vi "PreTell.vi"(8 "TellOriginEnum":T1, 9 "ListenerAlias":string, 10 "Message":refnum<class "Msg.lvclass">, 11 "Actor":refnum<class "Actor.lvclass">) -> (2 "Message":refnum<class "Msg.lvclass">)   [LabVIEW 2020, in "jettl.lvlib"]
uses:
  jettl.lvlib
  Origin.ctl
  Lifecycle.ctl
  Metadata.ctl
  Actor/Actor.lvclass
  Msg/Msg.lvclass
  Metadata/Metadata.lvclass
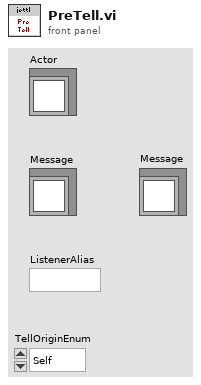
[diagram p1: front panel]
types:
  T1 = typedef "jettl.lvlib/Origin.ctl" = enum16{"Self", "Parent", "Child"}
  T2 = typedef "jettl.lvlib/Metadata.ctl" = cluster{"ListenerAlias":string, "TellerAlias":string, "Lifecycle":T3, "Origin":T1, "AbsoluteTime":timestamp, "RelativeTime":dbl, "Metadata":refnum<class "Metadata.lvclass">}
  T3 = typedef "jettl.lvlib/Lifecycle.ctl" = enum16{"Initializing", "SettingUp", "Starting", "Running", "Stopping", "TearingDown", "Terminated"}
  T4 = typedef "jettl.lvlib/Base.ctl" = cluster{"Lifecycle":T3, "SelfUnified":T5, "ParentUnified":T5, "ChildUnifiedMap":T7}
  T5 = typedef "jettl.lvlib/Unified.ctl" = cluster{"Alias":string, "MsgSet":T6, "Root":bool, "Leaf":bool, "MsgDVREvent":refnum<user-event>, "EventRegRef":refnum<event-registration>, "PreSetupQueue":refnum<queue>, "BeginSetupQueue":refnum<queue>, "PostSetupQueue":refnum<queue>, "VIRef":refnum<vi>, "DestroyQueue":refnum<queue>}
  T6 = typedef "jettl.lvlib/MsgSet.ctl" = set{refnum<class "Msg.lvclass">}
  T7 = typedef "jettl.lvlib/ChildUnifiedMap.ctl" = map{string, T5}
  T8 = typedef "jettl.lvlib/LifecycleEnum.ctl" = enum16{"Initializing", "SettingUp", "Starting", "Running", "Stopping", "TearingDown", "Terminated", "Abort"}
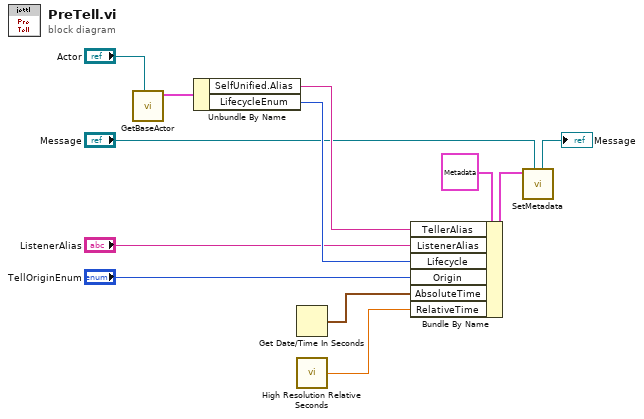
[diagram p0: block diagram]
diagram:
  n1 = call-dynamic "GetBaseActor.vi"("Actor"="Actor") -> ("BaseActor"=w12:T4)  [unwired: 10 in]
  n2 = Unbundle By Name(w12) -> ("SelfUnified.Alias"=w3:string, "LifecycleEnum"=w6:T8)
  n3 = Get Date/Time In Seconds() -> (seconds since 1Jan1904=w8:timestamp)
  n4 = call <vilib>:"High Resolution Relative Seconds.vi"() -> ("relative seconds"=w9:dbl)
  n5 = Bundle By Name(cluster=T2 {"ListenerAlias"="", "TellerAlias"="", "Lifecycle"=enum."Initializing", "Origin"=enum."Self", "AbsoluteTime"=timestamp(0 s since 1904-01-01), "RelativeTime"=0.0, "Metadata"=refnum} ("MessageMetadata"), "TellerAlias"=w3, "ListenerAlias"="ListenerAlias", "Lifecycle"=w6, "Origin"="TellOriginEnum", "AbsoluteTime"=w8, "RelativeTime"=w9) -> (w4:T2)
  n6 = call-dynamic "SetMetadata.vi"("Message"="Message", "MetadataCluster"=w4) -> ("Message"=→"Message":refnum<class "Msg.lvclass">)  [unwired: 9 in]
